vi "THzTime_SPEED_control(원본).vi"(1 "ESP300 Axis":i8=1, 2 "ESP300 Address":string="1", 4 "Lockin Address":string="12") -> ()   [LabVIEW 2010]
uses:
  <vilib>/Utility/file.llb/Write To Spreadsheet File (DBL).vi
panel:
  in  "Interdelay (ms)":dbl
  in  "pre delay(ms)":dbl=10.0
  out "Current deceleration":dbl=100.0
  in  "Acceleration":dbl
  out "Current acceleration":dbl=100.0
  in  "Set Acc":bool
  out "Current Velocity":dbl=25.0
  in  "Velocity":dbl
  in  "Set Velocity":bool
  in  "Reset Range":bool
  out "Boolean":bool
  out "MinValue":dbl=2.7285e-11 format="%#.3p"
  out "MinPosition":dbl=-2.240000009536743 format="%#.3f"
  out "Lock-in Y-Channel":dbl=2.5466e-11 format="%#.3p"
  out "Lock-in X-Channel":dbl=-5.457e-12 format="%#.3p"
  out "THz Time-domain Signal Wave":cluster{"x-axis":sgl[], "y-axis":dbl[]}(graph)={"x-axis"=[-3.0, -2.99, -2.98, -2.97, -2.96, -2.95, -2.94, -2.93, -2.92, -2.91, -2.9, -2.89, -2.88, -2.87, -2.86, -2.85, -2.84, -2.83, -2.82, -2.81, -2.8, -2.79, -2.78, -2.77, -2.76, -2.75, -2.74, -2.73, -2.72, -2.71, -2.7, -2.69, -2.68, -2.67, -2.66, -2.65, -2.64, -2.63, -2.6200001, -2.61, -2.6, -2.59, -2.58, -2.57, -2.56, -2.55, -2.54, -2.53, -2.52, -2.51, -2.5, -2.49, -2.48, -2.47, -2.46, -2.45, -2.44, -2.43, -2.42, -2.41, -2.4, -2.39, -2.38, -2.3700001, -2.3600001, -2.35, -2.34, -2.33, -2.32, -2.31, -2.3, -2.29, -2.28, -2.27, -2.26, -2.25, -2.24, -2.23, -2.22, -2.21, -2.2, -2.19, -2.18, -2.17, -2.16, -2.15, -2.14, -2.13, -2.1200001, -2.1100001, -2.1, -2.09, -2.08, -2.07, -2.06, -2.05, -2.04, -2.03, -2.02, -2.01, -2.0, -1.99, -1.98, -1.97, -1.96, -1.95, -1.94, -1.9300001, -1.9200001, -1.91, -1.9, -1.89, -1.88, -1.87, -1.86, -1.85, -1.84, -1.83, -1.82, -1.8100001, -1.8000001, -1.7900001, -1.78, -1.77, -1.76, -1.75, -1.74, -1.73, -1.72, -1.71, -1.7, -1.69, -1.6800001, -1.6700001, -1.6600001, -1.65, -1.64, -1.63, -1.62, -1.61, -1.6, -1.59, -1.58, -1.57, -1.5600001, -1.5500001, -1.5400001, -1.5300001, -1.52, -1.51, -1.5, -1.49, -1.48, -1.47, -1.46, -1.45, -1.44, -1.4300001, -1.4200001, -1.4100001, -1.4000001, -1.39, -1.38, -1.37, -1.36, -1.35, -1.34, -1.33, -1.32, -1.3100001, -1.3000001, -1.2900001, -1.2800001, -1.27, -1.26, -1.25, -1.24, -1.23, -1.22, -1.21, -1.2, -1.19, -1.1800001, -1.1700001, -1.1600001, -1.1500001, -1.14, -1.13, -1.12, -1.11, -1.1, -1.09, -1.08, -1.07, -1.0600001, -1.0500001, -1.0400001, -1.0300001, -1.0200001, -1.01, -1.0, -0.99000007], "y-axis"=[6.18461e-11, 6.18461e-11, 6.275559999999999e-11, 6.457460000000001e-11, 6.54841e-11, 6.63936e-11, 6.821255e-11, 7.00315e-11, 7.18505e-11, 7.36695e-11, 7.54885e-11, 7.6398e-11, 7.6398e-11, 7.8217e-11, 7.8217e-11, 7.8217e-11, 7.8217e-11, 7.8217e-11, 7.8217e-11, 7.8217e-11, 7.8217e-11, 7.8217e-11, 7.8217e-11, 7.8217e-11, 7.73075e-11, 7.6398e-11, 7.54885e-11, 7.4579e-11, 7.4579e-11, 7.4579e-11, 7.4579e-11, 7.4579e-11, 7.4579e-11, 7.4579e-11, 7.36695e-11, 7.276e-11, 7.276e-11, 7.276e-11, 7.18505e-11, 7.18505e-11, 7.276e-11, 7.18505e-11, 7.0941e-11, 7.0941e-11, 7.00315e-11, 6.9122e-11, 6.821255e-11, 6.63936e-11, 6.457460000000001e-11, 6.275559999999999e-11, 6.18461e-11, 6.18461e-11, 6.275559999999999e-11, 6.36651e-11, 6.63936e-11, 6.912205e-11, 7.275999999999999e-11, 7.6398e-11, 7.91265e-11, 8.09455e-11, 8.27645e-11, 8.3674e-11, 8.3674e-11, 8.3674e-11, 8.27645e-11, 8.09455e-11, 7.821699999999999e-11, 7.36695e-11, 6.821255e-11, 6.09366e-11, 5.54795e-11, 4.911295e-11, 4.2746500000000003e-11, 3.7289500000000003e-11, 3.2742e-11, 3.001355e-11, 2.7285e-11, 2.7285e-11, 2.819455e-11, 3.092305e-11, 3.4561000000000003e-11, 3.7289500000000003e-11, 3.9108499999999995e-11, 4.09275e-11, 4.45655e-11, 4.638445e-11, 5.00224e-11, 5.18414e-11, 5.36604e-11, 5.72985e-11, 5.82081e-11, 5.82081e-11, 5.82081e-11, 6.00271e-11, 6.09366e-11, 6.275559999999999e-11, 6.457460000000001e-11, 6.730305e-11, 7.00315e-11, 7.18505e-11, 7.36695e-11, 7.54885e-11, 7.6398e-11, 7.73075e-11, 7.8217e-11, 7.8217e-11, 7.8217e-11, 7.8217e-11, 7.8217e-11, 7.8217e-11, 7.8217e-11, 7.8217e-11, 7.8217e-11, 7.8217e-11, 7.8217e-11, 7.8217e-11, 7.91265e-11, 8.0036e-11, 8.0036e-11, 7.91265e-11, 7.8217e-11, 7.8217e-11, 7.8217e-11, 7.8217e-11, 7.91265e-11, 8.0036e-11, 8.0036e-11, 8.0036e-11, 8.09455e-11, 8.1855e-11, 8.09455e-11, 8.0036e-11, 7.91265e-11, 7.8217e-11, 7.8217e-11, 7.73075e-11, 7.54885e-11, 7.36695e-11, 7.18505e-11, 6.9122e-11, 6.73031e-11, 6.54841e-11, 6.457460000000001e-11, 6.36651e-11, 6.275559999999999e-11, 6.09366e-11, 6.00271e-11, 6.00271e-11, 6.00271e-11, 6.00271e-11, 6.09366e-11, 6.18461e-11, 6.18461e-11, 6.18461e-11, 6.275559999999999e-11, 6.36651e-11, 6.457460000000001e-11, 6.54841e-11, 6.457460000000001e-11, 6.36651e-11, 6.36651e-11, 6.36651e-11, 6.36651e-11, 6.36651e-11, 6.36651e-11, 6.36651e-11, 6.36651e-11, 6.36651e-11, 6.36651e-11, 6.36651e-11, 6.36651e-11, 6.36651e-11, 6.457460000000001e-11, 6.54841e-11, 6.457460000000001e-11, 6.457460000000001e-11, 6.54841e-11, 6.63936e-11, 6.73031e-11, 6.73031e-11, 6.9122e-11, 6.73031e-11, 6.821255e-11, 6.9122e-11, 6.9122e-11, 6.73031e-11, 6.821255e-11, 6.9122e-11, 6.9122e-11, 6.9122e-11, 6.9122e-11, 6.821255e-11, 6.73031e-11, 6.73031e-11, 6.73031e-11, 6.73031e-11, 6.73031e-11, 6.73031e-11, 6.63936e-11, 6.63936e-11, 6.54841e-11, 6.54841e-11]}
  in  "Autosave Directory for Long-term Average Scan":path=path "D:/KHA/20140828_reference/20140829/MAX1"
  out "Phase":cluster{"f0":dbl, "df":dbl, "magnitude":dbl[]}(graph)={"f0"=0.0, "df"=0.07425743035308216, "magnitude"=[0.0, 0.5430262224073249, -1.5115081089683766, 1.7772626748999498, -1.3535785331051065, -3.0255924301051373, 1.0617467642791563, -1.7528046215048894, -3.0245075812862505, 1.070509668872363, -1.1159718876864337, 2.987119361558609, 0.8316453969505877, 2.640508421043377, 0.9384552989713391, 2.9214790505897548, 3.0862999067619965, 1.4821111110084353, -0.009812840593746652, -2.886185847267045, 1.8281292234757007, -1.9632506198365165, 1.7986802942515163, -2.9100296826378456, 2.138205732046385, 0.7112165924710155, -2.3100505259605204, 0.2961041824562709, -1.0856579574789977, 2.6243227681827803, -2.579800649174383, -0.08999793591506308, 2.3320610301048266, -2.851407232095218, 1.4781561312800024, 1.4219006571187802, 1.0958693184455217, 2.391323419486901, 2.8799810415926164, 2.84488564721393, 1.635501401749418, -1.5731723920824747, 1.7193068993272027, 0.14486568153160087, -3.0895343822575168, 0.8905572023469569, 3.071997789642284, 2.9772092931422702, 1.4298576668959693, 2.3596614382380205, 0.03771580590821397, 2.8253495472955406, -1.8754571797660322, 2.5197616293101803, 0.6313140567621023, 0.5041655916505039, 1.1709004687927898, 2.3165329480728425, 2.181137256993364, 2.463406603924043, 1.2743204611978167, -2.125125263990236, -1.9243817713735893, -0.5414343998978727, 2.724418484956482, 1.5896882428075785, -0.6994818420158975, 2.3440945823246158, -2.1613168917281125, 2.4061082973570813, 1.3546841259026299, -2.4643381397140356, 0.4699394179047719, -3.0978241473705426, 1.7298779116894678, -0.2725008619561878, 1.9465714096650542, 1.230064042092765, 2.0364751589084245, 2.888769489510813, -1.4618251855550555, -2.0437438827709546, -2.0731237909445452, 2.4939264997201906, 1.7322437322624775, 2.740322990454104, 1.8481001050650303, -2.416624769728462, 2.78507832918226, 0.0031068433444392733, -2.4372275022639003, 1.04373155197689, 1.2095116956263916, 1.8951732814419298, 2.051959326610916, 2.463089830464577, -3.0823640934472905, -2.7947864385886505, -1.9951627739151572, -2.624931423227698, -2.439288880036958]}
  out "elapsed time":string=" 0 h   0 m  29 s"
  in  "OK Button":bool
  out "Data Type":string="outp ? 1"
  in  "Enum":enum16{"X", "Y", "Abs"}(ring)
  out "MaxValue":dbl=8.3674e-11 format="%#.3p"
  out "MaxPosition":dbl=-2.390000104904175 format="%#.3f"
  in  "Position":sgl=-15.0 format="%#.4f"
  in  "Find Max":bool
  in  "Set Position":bool
  in  "Save Data":bool
  in  "Draw":bool
  in  "Exit Program":bool
  out "Amplitude":cluster{"f0":dbl, "df":dbl, "magnitude":dbl[]}(graph)={"f0"=0.0, "df"=0.07425743035308216, "magnitude"=[6.785684183168313e-11, 1.865133249494546e-12, 7.015093269078534e-12, 4.870583726547154e-12, 3.147544049827258e-12, 4.00290874245221e-12, 3.278855913949389e-12, 2.06001316937915e-12, 2.4808684537999712e-12, 2.1766189198417383e-12, 9.367109018336555e-13, 1.1147800460570872e-12, 5.016275619742197e-13, 2.5268093192458076e-13, 2.0667810867362284e-13, 1.3852031200817767e-13, 1.6660740649803541e-13, 3.344138111014577e-13, 2.4910968701618634e-13, 8.495674278924137e-14, 1.6388152260015644e-13, 1.0591553556617101e-13, 1.37370465576575e-13, 1.5972149314608725e-13, 1.4057592588598159e-13, 3.8791757129205777e-14, 1.406089699290628e-13, 7.784010034048277e-14, 3.5922119595265765e-14, 1.2563751022281412e-13, 4.636148906830626e-14, 7.567862754592208e-14, 8.40057857660958e-14, 2.070704482137443e-14, 5.718704403756399e-14, 3.94065985935295e-14, 5.368395546248403e-14, 1.2827270368393742e-13, 6.905425225861492e-14, 4.3708190527670456e-14, 1.401600038739493e-14, 2.5565829763503863e-14, 9.084369637893239e-14, 4.6715303041465365e-14, 2.9307762038438304e-14, 8.8233419156545e-14, 6.687887978009298e-14, 2.9118906251587415e-14, 2.1731298815164244e-14, 6.179642006051064e-14, 7.483981136505485e-15, 5.185259239110594e-14, 3.6730092543975106e-14, 4.963825713758574e-14, 3.649899790222046e-14, 5.4295237051388733e-14, 8.346017151802908e-14, 2.888517003519212e-14, 6.203666590914844e-14, 6.41118241689492e-14, 3.6208519352709284e-14, 4.610237788015174e-14, 5.2095704441778304e-14, 5.795346869500378e-14, 1.1354905620046188e-14, 1.6430738458518083e-14, 3.368662729110748e-14, 2.3425157866612606e-14, 1.634630851403108e-14, 6.21143502913351e-14, 3.2057879572694906e-14, 2.6446384881008822e-14, 9.303366390581563e-15, 2.587806228859629e-14, 2.360848303533266e-14, 2.239212443289593e-14, 1.7710531108348354e-14, 2.0233938587896157e-14, 9.620857781698348e-15, 2.8456607293994056e-14, 2.323709473041354e-14, 1.4606070980626467e-14, 1.6767127252505727e-14, 2.3224857382870047e-14, 1.4731390104107788e-14, 4.072714869205643e-14, 4.60037180501932e-14, 4.004864790395104e-14, 5.855048769820165e-14, 2.0407288806914748e-14, 3.2531051493514047e-14, 3.2256575454405645e-14, 1.3847901783878021e-14, 3.6506129445661494e-14, 7.038305783719452e-15, 4.132026612397869e-14, 4.197578280883253e-14, 3.4309964316323095e-14, 3.0755227097706716e-14, 4.1349170484493553e-14, 1.429767862023511e-14]}
  in  "Short term \nAverage#":i8=2
  out "Numeric 2":i8=1
  in  "Long term \nAverage#":i8=1
  in  "Step":sgl=0.01 min=0 max=10000 format="%.3f"
  in  "End Position":sgl=-1.0 min=-75 max=75 format="%#.3f"
  in  "Start Position":sgl=-3.0 min=-75 max=75 format="%#.3f"
  # "This Program Run First (1) and then Run the Approach Program (2)"
  # "THz Experiment"
  # "Data"
  # "Auto-offset"
  # "Start Position (mm)"
  # "End Position (mm)"
  # "Step (mm)"
  # "Point Avg"
  # "Long Avg"
  # "Turn Number"
  # "mm"
  # "mm"
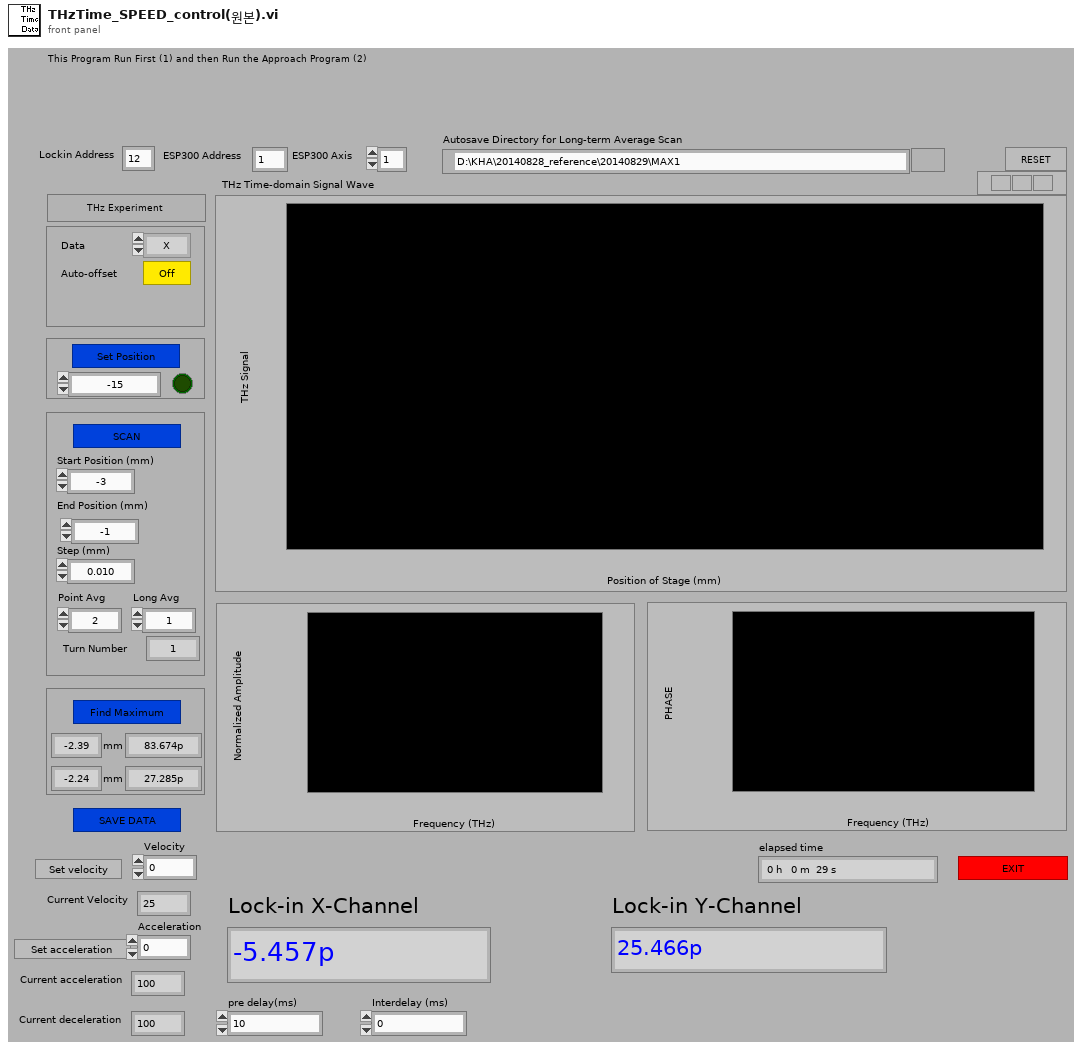
[diagram p1: front panel]
types:
  T1 = cluster{"Step Number":i32, "Step":sgl, "Start Position":sgl, "Time-out":i32, "Lockin Address":string, "Short term \nAverage#":i8, i32, "ESP300 Axis":i8, "Value":string, "pre delay(ms)":dbl, "Interdelay (ms)":dbl, "Autosave Directory for Long-term Average Scan":path}
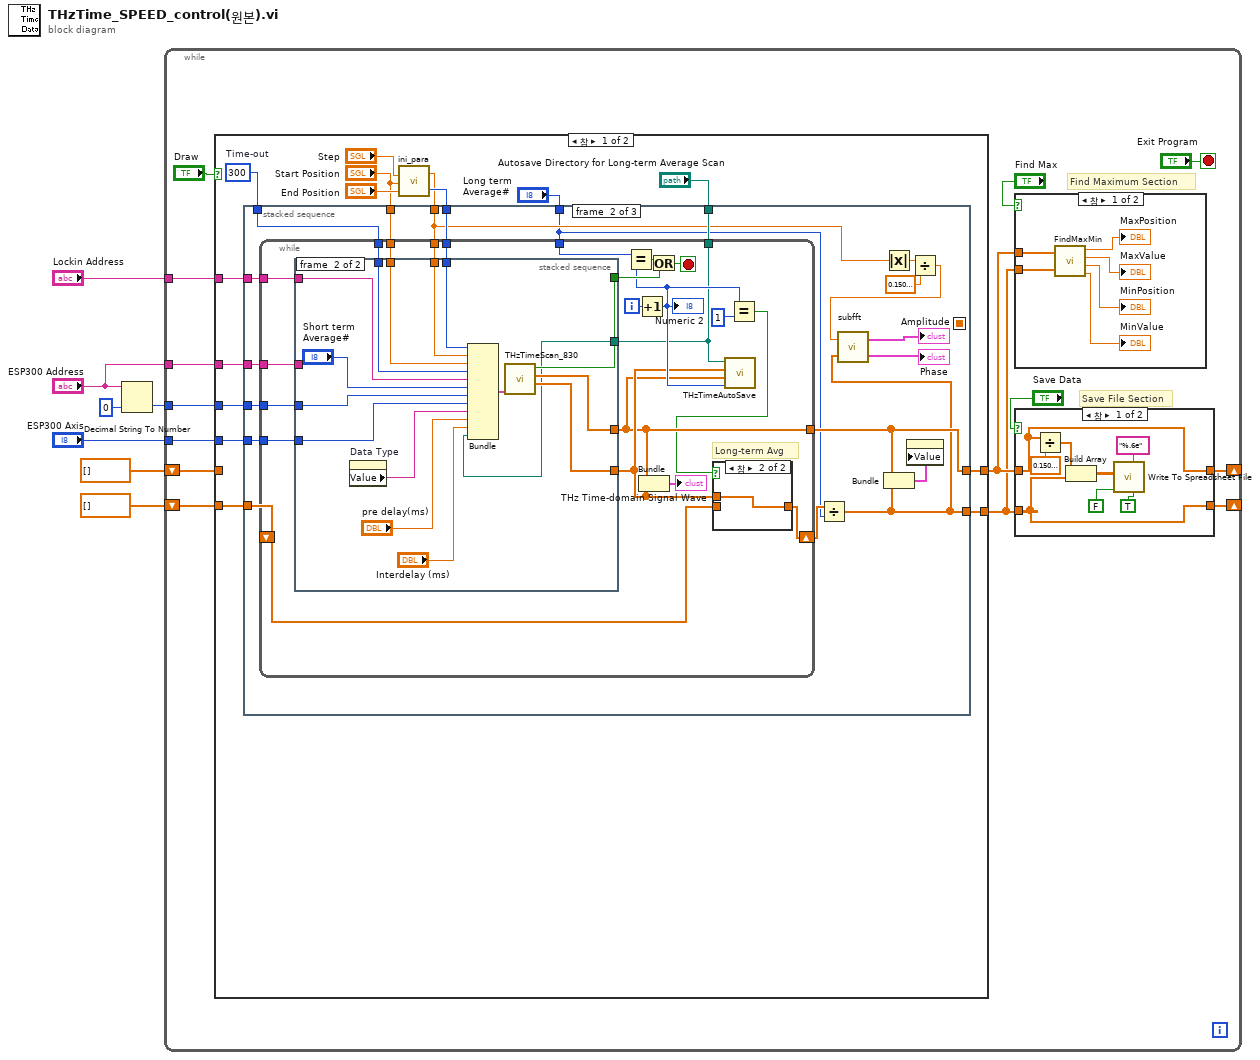
[diagram p0: block diagram]
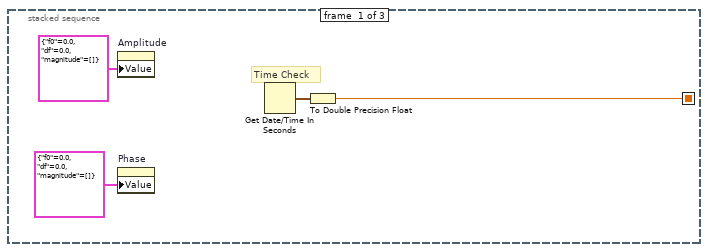
[diagram p4: hidden frame]
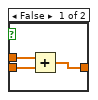
[diagram p5: hidden frame]
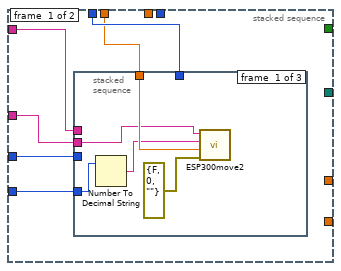
[diagram p6: hidden frame]
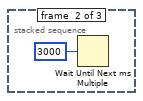
[diagram p7: hidden frame]
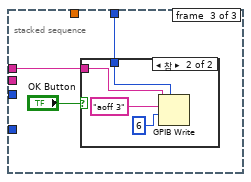
[diagram p8: hidden frame]
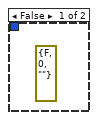
[diagram p9: hidden frame]
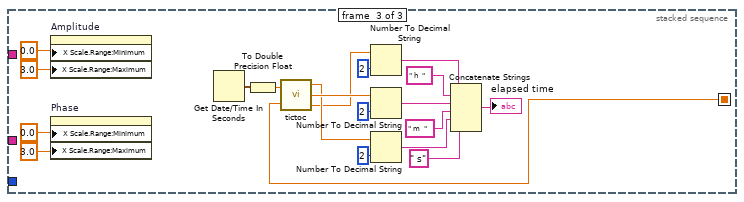
[diagram p10: hidden frame]
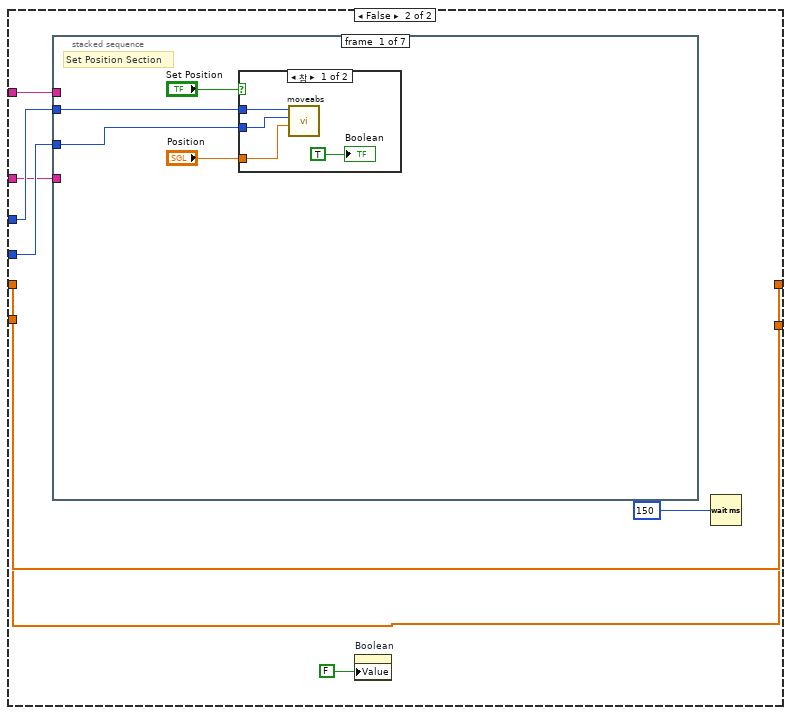
[diagram p11: hidden frame]
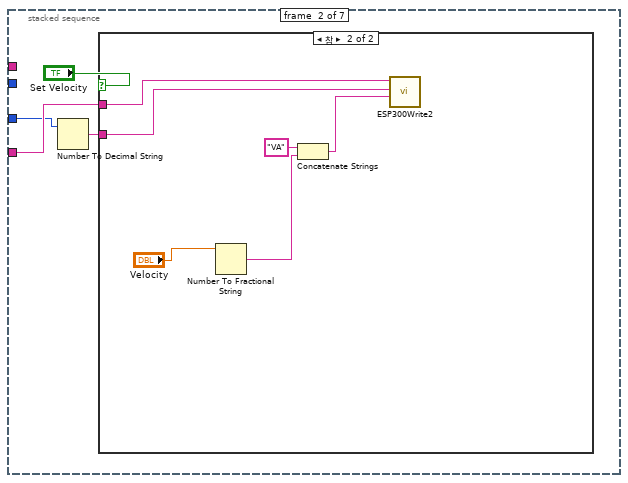
[diagram p13: hidden frame]
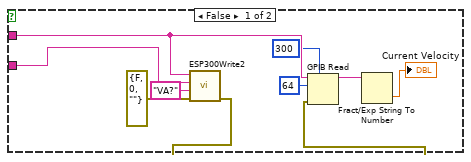
[diagram p14: hidden frame]
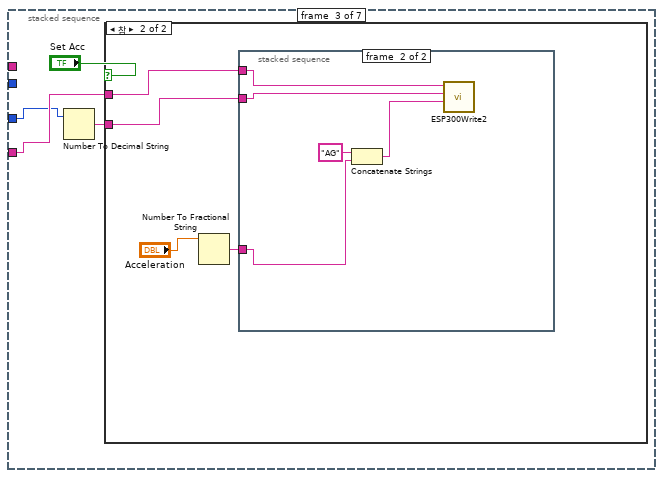
[diagram p15: hidden frame]
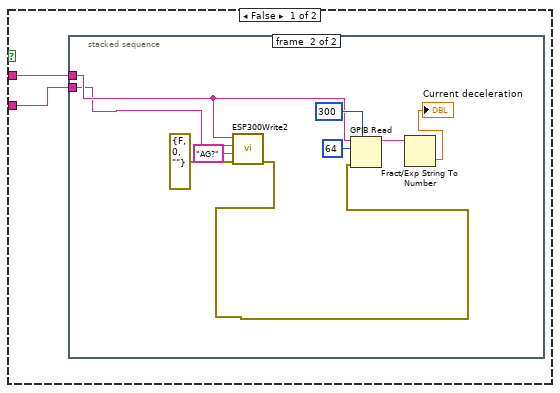
[diagram p16: hidden frame]
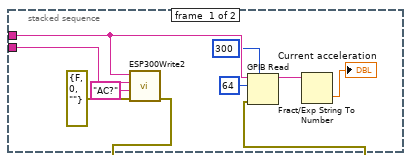
[diagram p17: hidden frame]
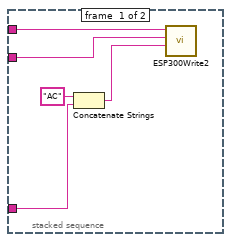
[diagram p18: hidden frame]
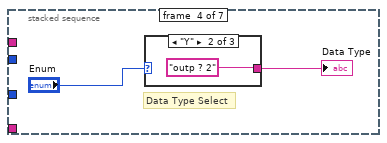
[diagram p19: hidden frame]
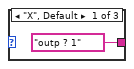
[diagram p20: hidden frame]
diagram:
  n1 = Decimal String To Number(string="ESP300 Address", default (0L)=0 ("default (0 I32)")) -> (number=w5:i32)  [unwired: 1 in, 1 out]
  n2 = while {
    tunnel: "ESP300 Axis" -> [w17]
    tunnel: "Lockin Address" -> [w16]
    tunnel: w5 -> [w15]
    shift-right: [w12] -> _
    shift-left: sgl[] [] -> [w14]
    shift-right: [w11] -> _
    shift-left: dbl[] [] -> [w13]
    tunnel: "ESP300 Address" -> [w8]
    stop <- "Exit Program" stop-if-true
    # "Save File Section"
    # "Find Maximum Section"
    n3 = case shown="참" "Draw" {
      tunnel: w16 -> [w52 w160]
      tunnel: w17 -> [w51 w165]
      tunnel: w15 -> [w50 w164]
      tunnel: [w41 w163] -> w10
      tunnel: [w40 w162] -> w9
      tunnel: w14 -> [_ w163]
      tunnel: w13 -> [w39 w162]
      tunnel: w8 -> [w38 w158]
      frame True {
        w48 = 300  # Time-out
        n4 = call "ini_para.vi"("End Position"="End Position", "Start Position"="Start Position", "Step"="Step") -> ("Step Number"=w45:i32, "Step"=w44:sgl)
        n5 = stacked-sequence {
          seq-local: [w54 _ _] -> [_ _ w138]
          tunnel: w52 -> [_ w76 _]
          tunnel: w48 -> [_ w75 _]
          tunnel: "Long term \nAverage#" -> [_ w58 _]
          tunnel: w51 -> [_ w74 _]
          tunnel: w50 -> [_ w73 _]
          tunnel: w45 -> [_ w71 _]
          tunnel: w44 -> [_ w63 _]
          tunnel: "Start Position" -> [_ w72 _]
          tunnel: "Autosave Directory for Long-term Average Scan" -> [_ w70 _]
          tunnel: [_ w61 _] -> w41
          tunnel: [_ w59 _] -> w40
          tunnel: w39 -> [_ w69 _]
          tunnel: w38 -> [_ w57 _]
          frame #0 {
            # "Time Check"
            n6 = property on="Amplitude" class="WFGraph (엄격한)"("Value"=cluster{"f0":dbl, "df":dbl, "magnitude":dbl[]} {"f0"=0.0, "df"=0.0, "magnitude"=[]} ("Spectrum")) -> ()  [unwired: 2 in, 2 out]
            n7 = property on="Phase" class="WFGraph (엄격한)"("Value"=cluster{"f0":dbl, "df":dbl, "magnitude":dbl[]} {"f0"=0.0, "df"=0.0, "magnitude"=[]} ("Spectrum")) -> ()  [unwired: 2 in, 2 out]
            n8 = Get Date/Time In Seconds() -> (seconds since 1Jan1904=w55:timestamp)
            n9 = To Double Precision Float(number=w55) -> (double precision float=w54:dbl)
          }
          frame #1 {
            n10 = while {
              tunnel: w58 -> [w96]
              tunnel: w75 -> [w97]
              tunnel: w76 -> [w98]
              tunnel: w74 -> [w92]
              tunnel: w73 -> [w91]
              tunnel: w72 -> [w90]
              tunnel: w63 -> [w89]
              tunnel: w71 -> [w88]
              tunnel: w70 -> [w77]
              shift-right: [w81] -> w60
              shift-left: w69 -> [w83]
              tunnel: [w80] -> w61
              tunnel: w57 -> [w78]
              i -> [w87]
              stop <- w95 stop-if-true
              # "Long-term Avg"
              n11 = stacked-sequence {
                tunnel: w98 -> [w108 w133]
                tunnel: w97 -> [w107 w134]
                tunnel: [_ w128] -> w93
                tunnel: w92 -> [w106 w130]
                tunnel: w91 -> [w105 w131]
                tunnel: w90 -> [w104 w135]
                tunnel: w89 -> [_ w136]
                tunnel: w88 -> [_ w137]
                tunnel: [_ w127] -> w80
                tunnel: [_ w126] -> w82
                tunnel: w78 -> [w103 _]
                tunnel: w77 -> [_ w122]
                frame #0 {
                  n12 = stacked-sequence {
                    tunnel: w108 -> [_ _ w116]
                    tunnel: w107 -> [_ _ w115]
                    tunnel: w106 -> [w110 _ _]
                    tunnel: w105 -> [_ _ _]
                    tunnel: w104 -> [w113 _ _]
                    tunnel: w103 -> [w111 _ _]
                    frame #0 {
                      n13 = Number To Decimal String(number=w110) -> (decimal integer string=w109:string)  [unwired: 1 in]
                      n14 = call "ESP300move2.vi"("ESP300 Address"=w111, "ESP300 Channel"=w109, "Target"=w113, "error in (no error) 2"=errorcluster {"status"=FALSE, "code"=0, "source"=""}) -> ()  [unwired: 6 in, 1 out]
                    }
                    frame #1 {
                      n15 = Wait Until Next ms Multiple(millisecond multiple=3000) -> ()  [unwired: 1 out]
                    }
                    frame #2 {
                      n16 = case shown="참" "OK Button" {
                        tunnel: w116 -> [_ w121]
                        tunnel: w115 -> [_ w119]
                        frame False {
                          (unwired) errorcluster {"status"=FALSE, "code"=0, "source"=""} ("error in")
                        }
                        frame True {
                          n17 = GPIB Write(0:w121, 1:"aoff 3" ("data"), 2:i16 6 ("mode (0)"), 4:w119) -> ()  [unwired: 1 in, 2 out]
                        }
                      }
                    }
                  }
                }
                frame #1 {
                  n18 = property on="Data Type" class="Str"() -> ("Value"=w129:string)  [unwired: 2 in, 2 out]
                  n19 = Bundle("Step Number"=w137, "Step"=w136, "Start Position"=w135, "Time-out"=w134, "Lockin Address"=w133, "Short term \nAverage#"="Short term \nAverage#", w131, "ESP300 Axis"=w130, "Value"=w129, "pre delay(ms)"="pre delay(ms)", "Interdelay (ms)"="Interdelay (ms)", "Autosave Directory for Long-term Average Scan"=w122) -> (w125:T1)  [unwired: 1 in]
                  n20 = call "THzTimeScan_830.vi"("input"=w125) -> ("loop stop"=w128:bool, "x-axis"=w127:sgl[], "y-axis"=w126:dbl[])  [unwired: 1 in]
                }
              }
              n21 = Increment(x=w87) -> (x+1=w85:i32)
              "Numeric 2" <- w85
              n22 = Equal?(x=w96, y=w85) -> (x = y?=w94:bool)
              n23 = Bundle("x-axis"=w80, "y-axis"=w82) -> (→"THz Time-domain Signal Wave":cluster{"x-axis":sgl[], "y-axis":dbl[]})  [unwired: 1 in]
              n24 = Or(x=w94, y=w93) -> (x .or. y?=w95:bool)
              n25 = call "THzTimeAutoSave.vi"("Numeric"=w85, "x-axis"=w80, "y-axis"=w82, "Autosave Directory for Long-term Average Scan"=w77) -> ()
              n26 = Equal?(x=w85, y=1) -> (x = y?=w79:bool)
              n27 = case shown="참" w79 {
                tunnel: w83 -> [w100 _]
                tunnel: w82 -> [w101 w102]
                tunnel: [w99 w102] -> w81
                frame False {
                  n28 = Add(x=w101, y=w100) -> (x+y=w99:dbl[])
                }
                frame True {
                }
              }
            }
            n29 = Divide(x=w60, y=w58) -> (x/y=w59:dbl[])
            n30 = Absolute Value(x=w63) -> (abs(x)=w64:sgl)
            n31 = Bundle("x-axis"=w61, w59) -> (w68:cluster{"x-axis":sgl[], dbl[]})  [unwired: 1 in]
            n32 = property on="THz Time-domain Signal Wave" class="XYGraph (엄격한)"("Value"=w68) -> ()  [unwired: 2 in, 2 out]
            n33 = Divide(x=w64, y=sgl 0.15) -> (x/y=w62:sgl)
            n34 = call "subfft.vi"("y-signal"=w59, "time step"=w62) -> ("Phase"=→"Phase":cluster{"f0":dbl, "df":dbl, "real part":dbl[]}, "Amplitude"=→"Amplitude":cluster{"f0":dbl, "df":dbl, "real part":dbl[]})
          }
          frame #2 {
            n35 = property on="Amplitude" class="WFGraph (엄격한)"("X Scale.Range:Minimum"=0.0 ("X Scale.Range:Maximum"), "X Scale.Range:Maximum"=3.0) -> ()  [unwired: 2 in, 2 out]
            n36 = property on="Phase" class="WFGraph (엄격한)"("X Scale.Range:Minimum"=0.0, "X Scale.Range:Maximum"=3.0) -> ()  [unwired: 2 in, 2 out]
            n37 = Get Date/Time In Seconds() -> (seconds since 1Jan1904=w143:timestamp)
            n38 = To Double Precision Float(number=w143) -> (double precision float=w142:dbl)
            n39 = call "tictoc.vi"("Value"=w142, "Value 2"=w138) -> ("sec"=w140:dbl, "min"=w141:dbl, "hour"=w139:dbl)
            n40 = Number To Decimal String(number=w139, width (-)=i16 2) -> (decimal integer string=w148:string)
            n41 = Number To Decimal String(number=w141, width (-)=i16 2) -> (decimal integer string=w154:string)
            n42 = Number To Decimal String(number=w140, width (-)=i16 2) -> (decimal integer string=w153:string)
            n43 = Concatenate Strings(w148, " h  " ("Substring"), w154, " m  " ("Substring"), w153, " s" ("Substring")) -> (→"elapsed time":string)
          }
        }
      }
      frame False {
        n44 = stacked-sequence {
          tunnel: w165 -> [w167 w175 w193 _ _ _ _]
          tunnel: w164 -> [w166 _ _ _ _ _ _]
          tunnel: w160 -> [_ _ _ _ w239 w243 _]
          tunnel: w158 -> [_ w176 w194 _ _ _ _]
          frame #0 {
            # "Set Position Section"
            n45 = case shown="참" "Set Position" {
              tunnel: "Position" -> [w173 _]
              tunnel: w167 -> [w172 _]
              tunnel: w166 -> [w170 _]
              frame True {
                n46 = call "moveabs.vi"("SetPosition"=w173, "EXP300 -3A Axis"=w172, "ESP300 -3A Add."=w170) -> ()  [unwired: 2 in]
                "Boolean" <- TRUE
              }
              frame False {
              }
            }
          }
          frame #1 {
            n47 = Number To Decimal String(number=w175) -> (decimal integer string=w174:string)  [unwired: 1 in]
            n48 = case shown="참" "Set Velocity" {
              tunnel: w176 -> [w183 w192]
              tunnel: w174 -> [w186 w191]
              frame False {
                n49 = call "ESP300Write2.vi"("error in (no error)"=errorcluster {"status"=FALSE, "code"=0, "source"=""}, "Command"="VA?", "ESP300 Channel"=w186, "ESP300 Address"=w183) -> ("error out"=w178:errorcluster)  [unwired: 3 in]
                n50 = GPIB Read(0:w183, 1:64 ("byte count"), 3:w178, 4:300 ("timeout ms (488.2 global)")) -> (5:w182:string)  [unwired: 1 in, 2 out]
                n51 = Fract/Exp String To Number(string=w182) -> (number=→"Current Velocity":dbl)  [unwired: 3 in, 1 out]
              }
              frame True {
                n52 = Number To Fractional String(number="Velocity") -> (F-format string=w189:string)  [unwired: 3 in]
                n53 = Concatenate Strings("VA" ("string"), w189) -> (w187:string)
                n54 = call "ESP300Write2.vi"("Command"=w187, "ESP300 Channel"=w191, "ESP300 Address"=w192) -> ()  [unwired: 4 in, 1 out]
              }
            }
          }
          frame #2 {
            n55 = Number To Decimal String(number=w193) -> (decimal integer string=w195:string)  [unwired: 1 in]
            n56 = case shown="참" "Set Acc" {
              tunnel: w194 -> [w197 w217]
              tunnel: w195 -> [w198 w220]
              frame False {
                n57 = stacked-sequence {
                  tunnel: w198 -> [w207 w210]
                  tunnel: w197 -> [w204 w211]
                  frame #0 {
                    n58 = call "ESP300Write2.vi"("error in (no error)"=errorcluster {"status"=FALSE, "code"=0, "source"=""}, "Command"="AC?", "ESP300 Channel"=w207, "ESP300 Address"=w204) -> ("error out"=w199:errorcluster)  [unwired: 3 in]
                    n59 = GPIB Read(0:w204, 1:64 ("byte count"), 3:w199, 4:300 ("timeout ms (488.2 global)")) -> (5:w203:string)  [unwired: 1 in, 2 out]
                    n60 = Fract/Exp String To Number(string=w203) -> (number=→"Current acceleration":dbl)  [unwired: 3 in, 1 out]
                  }
                  frame #1 {
                    n61 = call "ESP300Write2.vi"("error in (no error)"=errorcluster {"status"=FALSE, "code"=0, "source"=""}, "Command"="AG?", "ESP300 Channel"=w210, "ESP300 Address"=w211) -> ("error out"=w209:errorcluster)  [unwired: 3 in]
                    n62 = GPIB Read(0:w211, 1:64 ("byte count"), 3:w209, 4:300 ("timeout ms (488.2 global)")) -> (5:w214:string)  [unwired: 1 in, 2 out]
                    n63 = Fract/Exp String To Number(string=w214) -> (number=→"Current deceleration":dbl)  [unwired: 3 in, 1 out]
                  }
                }
              }
              frame True {
                n64 = Number To Fractional String(number="Acceleration") -> (F-format string=w218:string)  [unwired: 3 in]
                n65 = stacked-sequence {
                  tunnel: w217 -> [w225 w228]
                  tunnel: w220 -> [w224 w227]
                  tunnel: w218 -> [w223 w226]
                  frame #0 {
                    n66 = Concatenate Strings("AC" ("string"), w223) -> (w221:string)
                    n67 = call "ESP300Write2.vi"("Command"=w221, "ESP300 Channel"=w224, "ESP300 Address"=w225) -> ()  [unwired: 4 in, 1 out]
                  }
                  frame #1 {
                    n68 = Concatenate Strings("AG" ("string"), w226) -> (w229:string)
                    n69 = call "ESP300Write2.vi"("Command"=w229, "ESP300 Channel"=w227, "ESP300 Address"=w228) -> ()  [unwired: 4 in, 1 out]
                  }
                }
              }
            }
          }
          frame #3 {
            # "Data Type Select"
            n70 = case shown="\"Y\"" "Enum" {
              tunnel: ["outp ? 1" "outp ? 2" "outp ? 3"] -> w232
              frame "X", Default {
              }
              frame "Y" {
              }
              frame "Abs" {
              }
            }
            "Data Type" <- w232
          }
          frame #4 {
            n71 = call "readdata_830.vi"("Command"="outp ? 1", "timeout"=200, "Lockin Address"=w239) -> ("Data"=→"Lock-in X-Channel":dbl)  [unwired: 1 in, 1 out]
          }
          frame #5 {
            n72 = call "readdata_830.vi"("Command"="outp ? 2", "timeout"=200, "Lockin Address"=w243) -> ("Data"=→"Lock-in Y-Channel":dbl)  [unwired: 1 in, 1 out]
          }
          frame #6 {
            n73 = case shown="참" "Reset Range" {
              frame False {
              }
              frame True {
                n74 = property on="Start Position" class="DigNum (엄격한)"() -> ("Value"=w246:sgl)  [unwired: 2 in, 2 out]
                n75 = property on="End Position" class="DigNum (엄격한)"() -> ("Value"=w245:sgl)  [unwired: 2 in, 2 out]
                n76 = property on="THz Time-domain Signal Wave" class="XYGraph (엄격한)"("X Scale.Range:Minimum"=w246, "X Scale.Range:Maximum"=w245) -> ()  [unwired: 2 in, 2 out]
              }
            }
          }
        }
        n77 = property on="Boolean" class="Bool (엄격한)"("Value"=FALSE ("Boolean")) -> ()  [unwired: 2 in, 2 out]
        n78 = Wait (ms)(milliseconds to wait=u32 150) -> ()  [unwired: 1 out]
      }
    }
    n79 = case shown="참" "Find Max" {
      tunnel: w10 -> [w37 _]
      tunnel: w9 -> [w36 _]
      frame True {
        n80 = call "FindMaxMin.vi"("x-axis"=w37, "y-axis"=w36) -> ("MaxPosition"=→"MaxPosition":dbl, "MaxValue"=→"MaxValue":dbl, "MinPosition"=→"MinPosition":dbl, "MinValue"=→"MinValue":dbl)
      }
      frame False {
      }
    }
    n81 = case shown="참" "Save Data" {
      tunnel: w10 -> [w22 w31]
      tunnel: w9 -> [w23 w30]
      tunnel: [w22 w31] -> w12
      tunnel: [w23 w30] -> w11
      frame True {
        n82 = Divide(x=w22, y=sgl 0.15) -> (x/y=w24:sgl[])
        n83 = Build Array(w24, w23) -> (w26:dbl[][])
        n84 = call-poly <vilib>:"Write To Spreadsheet File.vi"("transpose? (no:F)"=TRUE ("transpose?\n(no:F)"), "format (%.3f)"="%.6e", "append to file? (new file:F)"=FALSE ("append to file?\n(new file:F)"), "2D data"=w26) -> ()  [unwired: 4 in, 1 out]
      }
      frame False {
      }
    }
  }
